vi "New Interface Error.vi"(5 "error source class name":string, 7 "error source vi name":string, 11 "error":T1) -> (1 "new offset":i32, 3 "error out":errorcluster)   [LabVIEW 2017, in "DSF Core.lvlib" / "Interface.lvclass"]
uses:
  Interface.lvclass
  Errors.ctl
  Shared/Constants/Engine Library Name.vi
  <vilib>/NI/Memory Manager/VIs/New Error Cluster Constant (512B).vi
  <vilib>/NI/Memory Manager/Static Error Handling.lvlib
  DSF Core.lvlib
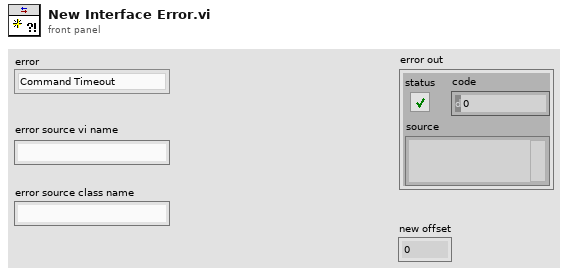
[diagram p1: front panel]
types:
  T1 = typedef "DSF Core.lvlib/Interface.lvclass/Errors.ctl" = enum16{"Command Timeout", "Response Timeout", "Error Timeout", "Invalid Response", "Invalid Response Parameters"}
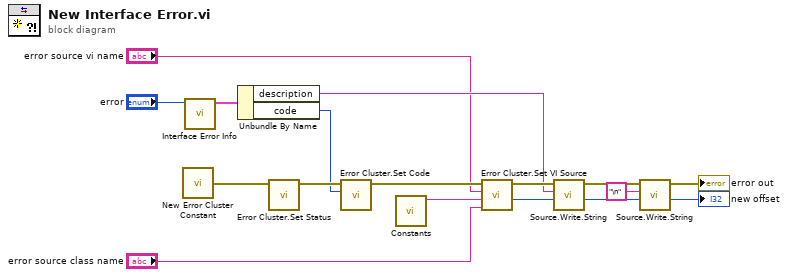
[diagram p0: block diagram]
diagram:
  n1 = call-poly <vilib>:"New Error Cluster Constant.vi"() -> ("error out"=w16:errorcluster)  [unwired: 1 in]
  n2 = call "Interface Error Info.vi"("error"="error") -> ("error info"=w14:cluster{"code":i32, "description":string})  [unwired: 10 in]
  n3 = Unbundle By Name(w14) -> ("description"=w8:string, "code"=w13:i32)
  n4 = call <vilib>:"Error Cluster.Set Status.vi"("error in"=w16) -> ("error out"=w15:errorcluster)  [unwired: 10 in]
  n5 = call <vilib>:"Error Cluster.Set Code.vi"("code"=w13, "error in"=w15) -> ("error out"=w12:errorcluster)  [unwired: 9 in]
  n6 = call-poly "Constants.vi"() -> ("Engine Library Name"=w11:string)  [unwired: 11 in]
  n7 = call <vilib>:"Error Cluster.Set VI Source.vi"("class name (\"\")"="error source class name", "library name (\"\")"=w11, "vi name"="error source vi name", "error in"=w12) -> ("new offset"=w9:i32, "error out"=w10:errorcluster)  [unwired: 6 in]
  n8 = call <vilib>:"Source.Write.String.vi"("offset"=w9, "string"=w8, "error in"=w10) -> ("new offset"=w5:i32, "error out"=w7:errorcluster)  [unwired: 7 in]
  n9 = call <vilib>:"Source.Write.String.vi"("offset"=w5, "string"="\n", "error in"=w7) -> ("new offset"=→"new offset":i32, "error out"=→"error out":errorcluster)  [unwired: 7 in]
